vi "Sequence Get RPM.vi"(11 "Sequencer Data Context IN":T1={"Sequencer State"=enum."Idle", "Event Timeout"=-1, "Current Index"=0, "Sequence Timeout"=0, "Turbine RPM Array"=[], "Pump RPM Array"=[], "Duration (Seconds) Array"=[]}) -> (3 "Sequencer Data Context OUT":T1={"Sequencer State"=enum."Idle", "Event Timeout"=-1, "Current Index"=0, "Sequence Timeout"=0, "Turbine RPM Array"=[], "Pump RPM Array"=[], "Duration (Seconds) Array"=[]}, 4 "Pump RPM":i16, 6 "Turbine RPM":i16)   [LabVIEW 2024, in "Auto Modo.lvlib"]
uses:
  Auto Modo.lvlib
  Sequencer State.ctl
  Sequencer Data Context.ctl
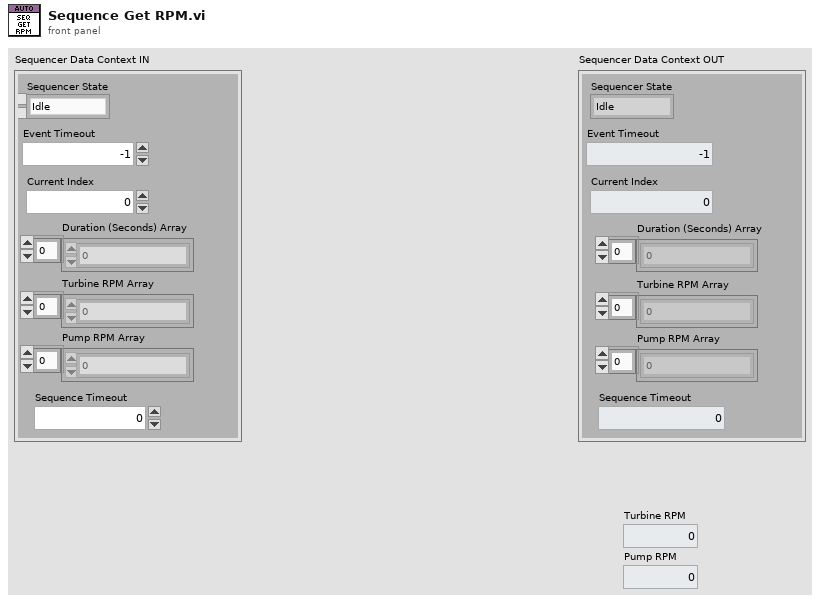
[diagram p1: front panel]
types:
  T1 = typedef "Auto Modo.lvlib/Sequencer Data Context.ctl" = cluster{"Sequencer State":T2, "Event Timeout":i32, "Current Index":i32, "Sequence Timeout":i32, "Turbine RPM Array":dbl[], "Pump RPM Array":dbl[], "Duration (Seconds) Array":dbl[]}
  T2 = typedef "Auto Modo.lvlib/Sequencer State.ctl" = enum16{"Idle", "Clear Drive Fault", "Check Drive Fault", "Set Ready to Switch ON", "Check Ready to Switch ON", "Enable Operation", "Check Enable Operation", "Set Drive RPM", "Final"}
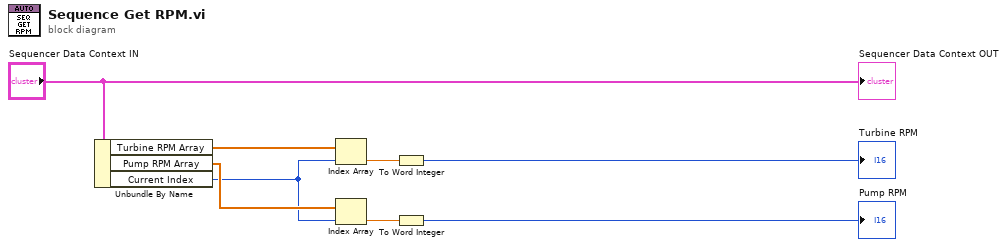
[diagram p0: block diagram]
diagram:
  n1 = Unbundle By Name("Sequencer Data Context IN") -> ("Turbine RPM Array"=w7:dbl[], "Pump RPM Array"=w6:dbl[], "Current Index"=w5:i32)
  n2 = Index Array(array=w7, index=w5) -> (element=w4:dbl)
  n3 = Index Array(array=w6, index=w5) -> (element=w3:dbl)
  n4 = To Word Integer(number=w4) -> (16bit integer=→"Turbine RPM":i16)
  n5 = To Word Integer(number=w3) -> (16bit integer=→"Pump RPM":i16)
  "Sequencer Data Context OUT" <- "Sequencer Data Context IN"
